vi "DSF.Engine.Execution.Builder.Get Execution Settings.vi"(8 "error in (no error)":errorcluster, 11 "Builder in":refnum<class "DSF.Engine.Execution.Builder.lvclass">) -> (0 "error out":errorcluster, 2 "Execution Settings":T1 {"Response Timeout" format="%d ms"; "Command Timeout" format="%d ms"}, 3 "Builder out":refnum<class "DSF.Engine.Execution.Builder.lvclass">)   [LabVIEW 2016, in "DSF.Engine.lvlib" / "DSF.Engine.Execution.Builder.lvclass"]
uses:
  Builder/DSF.Engine.Execution.Builder.lvclass
  DSF.Engine.Execution.Builder.Execution Settings.ctl
  Builder/DSF.Engine.Execution.Builder.lvclass/DSF.Engine.Execution.Builder.ctl
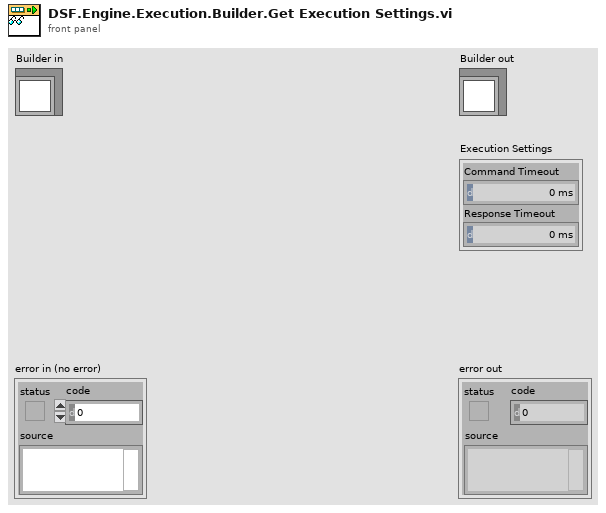
[diagram p1: front panel]
types:
  T1 = typedef "DSF.Engine.lvlib/DSF.Engine.Execution.Builder.lvclass/DSF.Engine.Execution.Builder.Execution Settings.ctl" = cluster{"Command Timeout":i32, "Response Timeout":i32}
  T2 = typedef "DSF.Engine.lvlib/DSF.Execution.Builder.lvclass/DSF.Engine.Execution.Builder.Execution Settings.ctl" = cluster{"Command Timeout":i32, "Response Timeout":i32}
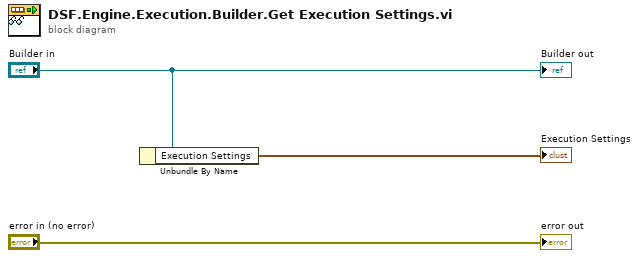
[diagram p0: block diagram]
diagram:
  n1 = Unbundle By Name("Builder in") -> ("Execution Settings"=→"Execution Settings":T2)
  "error out" <- "error in (no error)"
  "Builder out" <- "Builder in"
